vi "Main.vi"(11 "Module Admin":refnum<class "Delacor_lib_QMH_Module Admin.lvclass">) -> ()   [LabVIEW 2020, in "Molde.lvlib"]
doc: "This template is based off of the Queued Message Handler design pattern and the Queued Message Handler project template that ships with LabVIEW.\n\nThe main difference is that the queue is private to this module and communication between modules is performed via Broadcast and Request events.\n\nRequest events are wrapped in public API methods and are handled in the Event Handling Loop (EHL) of this VI. Any module can register for Broadcast events sent by this module. The EHL generates messages based on user interface actions.\n\nThe Message Handling Loop (MHL) processes messages generated by the EHL, or by other messages. The messages are string values, so new messages can be added easily to the Message Cases case structure in the MHL. Each message cluster can also provide an optional value for Message Data, which is a variant that can be converted to whatever message-specific data is required.\n_____\nBased on Delacor QMH Project Template 5.0.0.82."
uses:
  Molde.lvlib
  <vilib>/Delacor/Delacor QMH/Libraries/Module Admin_class/Delacor_lib_QMH_Module Admin.lvclass
  Module Data--cluster.ctl
  <vilib>/Delacor/Delacor QMH/Libraries/Message Queue_class/Delacor_lib_QMH_Message Queue.lvclass/Delacor_lib_QMH_Message Queue.ctl
  Stop Argument--cluster.ctl
  <vilib>/Delacor/Delacor QMH/Libraries/Module Admin_class/Delacor_lib_QMH_Module Admin.lvclass/Delacor_lib_QMH_Module Admin.ctl
  <vilib>/Utility/miscctls.llb/LVPointTypeDef.ctl
  <vilib>/Delacor/Delacor QMH/Libraries/Message Queue_class/Delacor_lib_QMH_Enqueue Message (Single).vi
  <vilib>/Delacor/Delacor QMH/Libraries/Module Admin_class/Delacor_lib_QMH_Get External Launch.vi
  <vilib>/Utility/error.llb/Error Cluster From Error Code.vi
  <vilib>/ErrorRing/Error Ring.xnode
  <vilib>/Delacor/Delacor QMH/Libraries/Message Queue_class/Delacor_lib_QMH_Message Queue.lvclass
  Numpad/Numpad.lvlib
panel:
  in  "Insertar Subpanel NumPad":bool
  in  "Simulate MHL Error":bool
  in  "Simulate EHL Error":bool
  out "error out":errorcluster
  out "Status":string
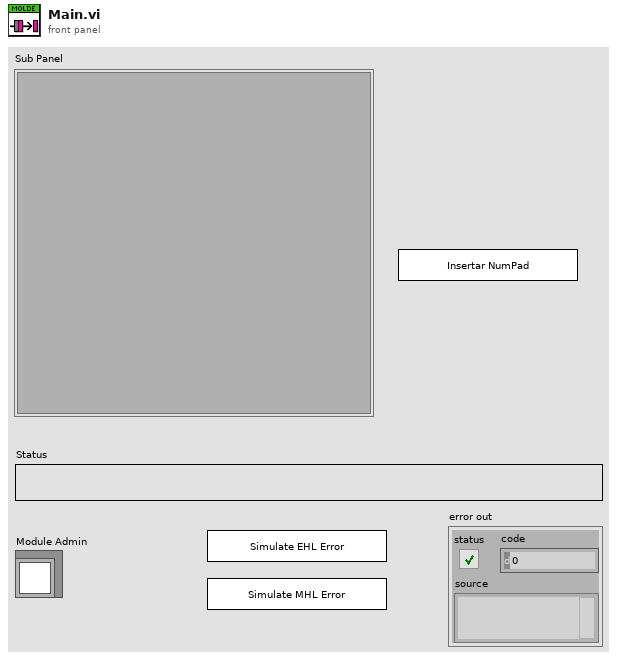
[diagram p1: front panel]
types:
  T1 = typedef "Molde.lvlib/Request Events--cluster.ctl" = cluster{"Stop Module":refnum<user-event>, "Show Panel":refnum<user-event>, "Hide Panel":refnum<user-event>, "Get Module Execution Status":refnum<user-event>, "Show Diagram":refnum<user-event>}
  T2 = typedef "Numpad.lvlib/Broadcast Events--cluster.ctl" = cluster{"Module Did Init":refnum<user-event>, "Status Updated":refnum<user-event>, "Error Reported":refnum<user-event>, "Module Did Stop":refnum<user-event>, "Update Module Execution Status":refnum<user-event>}
  T3 = typedef "Molde.lvlib/Module Data--cluster.ctl" = cluster{"Status":string}
  T4 = enum32{"invalid lock state", "Not Locked", "Locked (No Password)", "Password-protected"}
  T5 = typedef "Molde.lvlib/Stop Argument--cluster.ctl" = cluster{"Origin":string, "Exit via Stop Module Req?":bool, "Wait for Module to stop?":bool}
  T6 = typedef "LVPointTypeDef.ctl" = cluster{"Horizontal":i16, "Vertical":i16}
  T7 = enum32{"Invalid", "Standard", "Closed", "Hidden", "Minimized", "Maximized"}
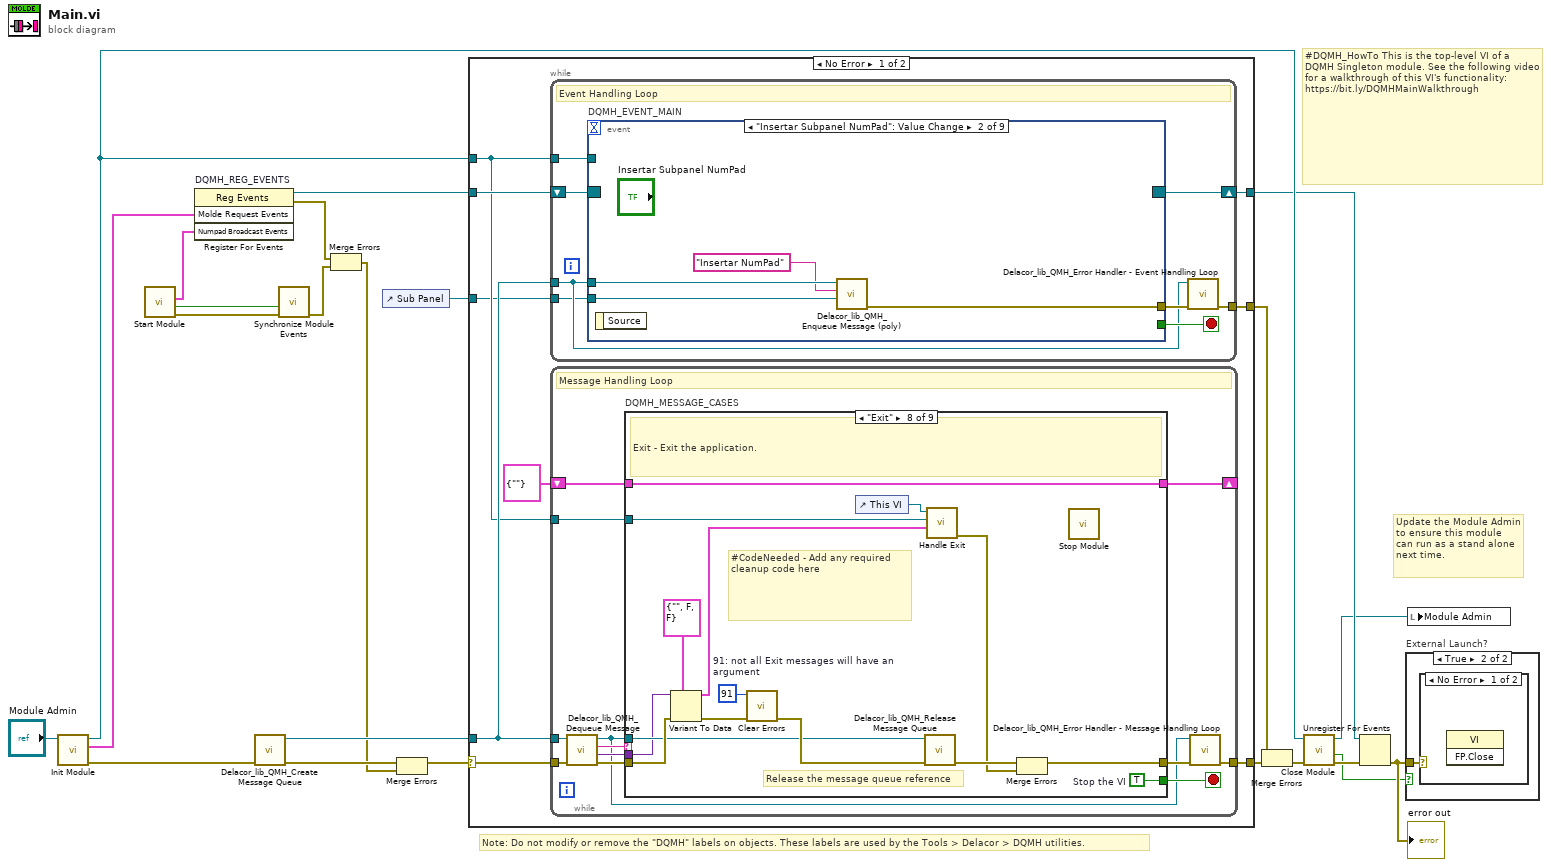
[diagram p0: block diagram]
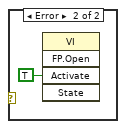
[diagram p3: hidden frame]
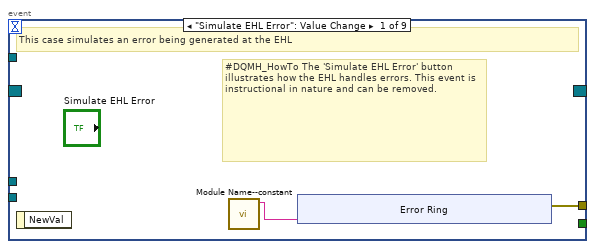
[diagram p4: hidden frame]
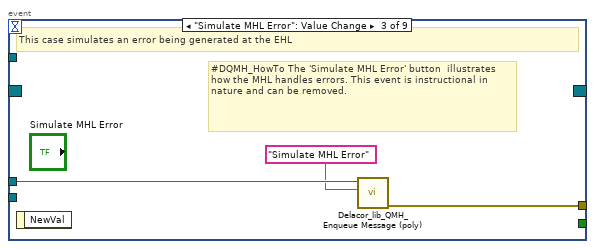
[diagram p5: hidden frame]
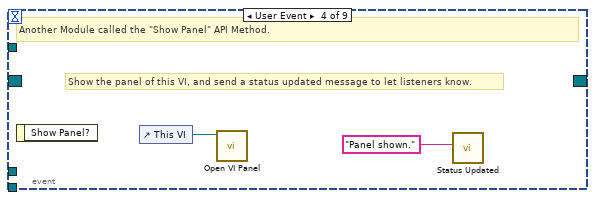
[diagram p6: hidden frame]
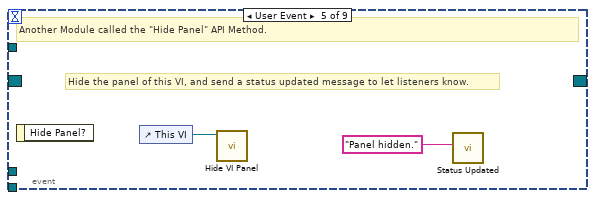
[diagram p7: hidden frame]
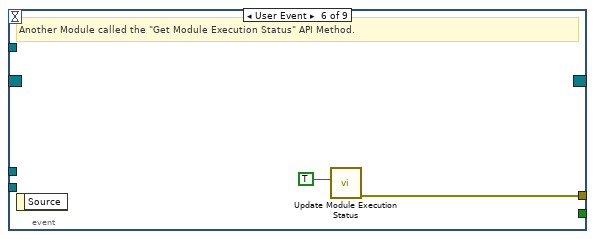
[diagram p8: hidden frame]
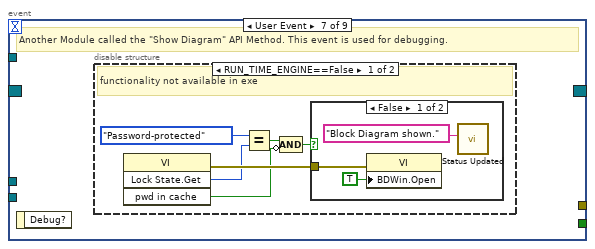
[diagram p9: hidden frame]
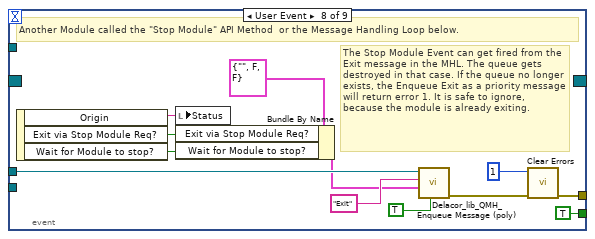
[diagram p12: hidden frame]
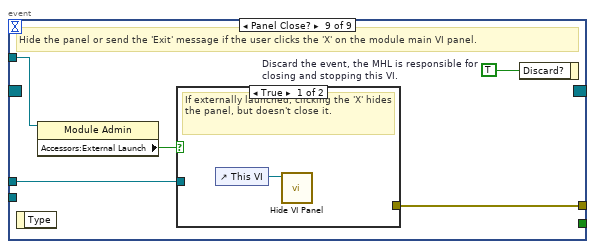
[diagram p13: hidden frame]
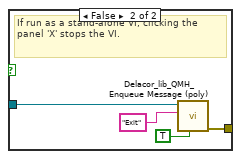
[diagram p14: hidden frame]
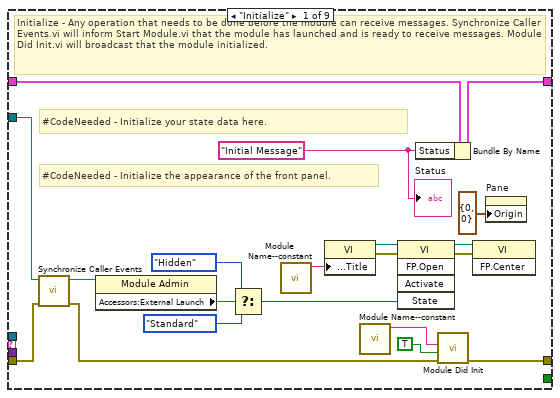
[diagram p15: hidden frame]
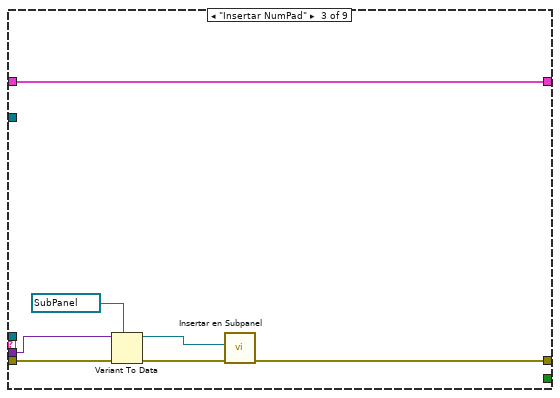
[diagram p17: hidden frame]
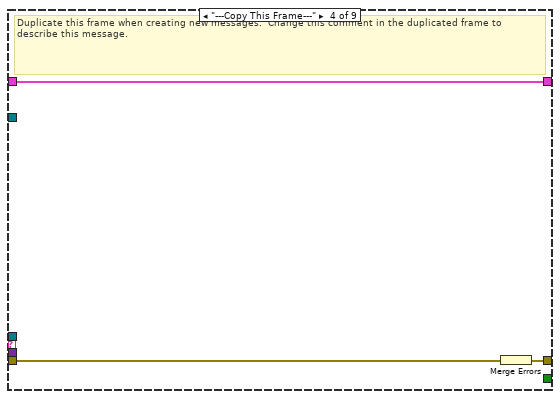
[diagram p18: hidden frame]
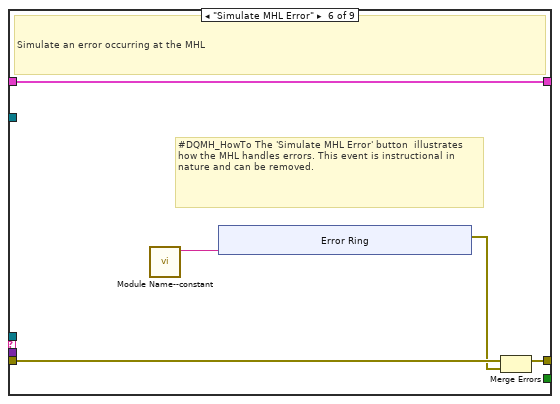
[diagram p20: hidden frame]
diagram:
  # "#DQMH_HowTo This is the top-level VI of a DQMH Singleton module. See the following video for a walkthrough of this VI's functionality: https://bit.ly/DQMHMainWalkthrough"
  # "Note: Do not modify or remove the \"DQMH\" labels on objects. These labels are used by the Tools > Delacor > DQMH utilities."
  # "Update the Module Admin to ensure this module can run as a stand alone next time."
  n1 = call "Init Module.vi"("Singleton Module Admin in"="Module Admin") -> ("error out"=w22:errorcluster, "Molde Request Events"=w12:T1, "Singleton Module Admin out"=w15:refnum<class "Delacor_lib_QMH_Module Admin.lvclass">)  [unwired: 8 in]
  n2 = call "Start Module.vi"() -> ("error out"=w5:errorcluster, "Wait for Event Sync?"=w7:bool, "Numpad Broadcast Events"=w6:T2)  [unwired: 8 in, 1 out]
  n3 = register-events "DQMH_REG_EVENTS"(w12, w6) -> (reference out=w13:refnum<event-registration>, error out=w4:errorcluster)  [unwired: 2 in]
  n4 = call <vilib>:"Delacor_lib_QMH_Create Message Queue.vi"("error in (no error)"=w22) -> ("error out"=w17:errorcluster, "Message Queue"=w11:refnum<class "Delacor_lib_QMH_Message Queue.lvclass">)  [unwired: 9 in]
  n5 = call "Synchronize Module Events.vi"("error in (no error)"=w5, "Wait for Event Sync?"=w7) -> ("error out"=w3:errorcluster)  [unwired: 9 in]
  n6 = Merge Errors(w4, w3) -> (w2:errorcluster)
  n7 = control-ref of="Sub Panel"() -> (w1:refnum<vi>)
  n8 = Merge Errors(w17, w2) -> (w16:errorcluster)
  n9 = case shown="No Error" w16 {
    selector: w16 -> [w30 w200]
    tunnel: [w32 w199] -> w23
    tunnel: [w29 w205] -> w14
    tunnel: w13 -> [w27 w205]
    tunnel: w11 -> [w26 w198]
    tunnel: [w31 _] -> w20
    tunnel: w15 -> [w25 w201]
    tunnel: w1 -> [w24 _]
    frame No Error {
      n10 = while {
        tunnel: w26 -> [w34]
        shift-right: [w37] -> w29
        shift-left: w27 -> [w38]
        tunnel: [w39] -> w31
        tunnel: w25 -> [w35]
        tunnel: w24 -> [w33]
        stop <- w36 stop-if-true
        # "Event Handling Loop"
        n11 = event "DQMH_EVENT_MAIN" shown="[1] \"Insertar Subpanel NumPad\": Value Change" {
          selector: w38 -> [_ _ _ _ _ _ _ _ _]
          dyn-events: [_ _ _ _ _ _ _ _ _] -> w37
          timeout: _ -> [_ _ _ _ _ _ _ _ _]
          tunnel: [_ _ _ _ _ _ _ TRUE ("Discard?") _] -> w36
          tunnel: w34 -> [_ w53 w55 _ _ _ _ w79 w86]
          tunnel: [w42 w50 w56 _ _ w62 _ w82 w88] -> w40
          tunnel: w35 -> [_ _ _ _ _ _ _ _ w85]
          tunnel: w33 -> [_ w52 _ _ _ _ _ _ _]
          event "Simulate EHL Error": Value Change {
            # "#DQMH_HowTo The 'Simulate EHL Error' button  illustrates how the EHL handles errors. This event is instructional in nature and can be removed."
            # "This case simulates an error being generated at the EHL"
            n12 = event-data() -> ()  [unwired: 1 in, 1 out]
            n13 = call "Module Name--constant.vi"() -> ("Module Name"=w41:string)  [unwired: 11 in]
            n14 = xnode "Error Ring"("parameter 0"=w41) -> ("error out"=w42:errorcluster)
          }
          event "Insertar Subpanel NumPad": Value Change {
            n15 = event-data() -> ()  [unwired: 1 in, 1 out]
            n16 = call-poly <vilib>:"Delacor_lib_QMH_Enqueue Message (poly).vi"("Message Data"=w52, "Message"="Insertar NumPad", "Message Queue in"=w53) -> ("error out"=w50:errorcluster)  [unwired: 7 in, 1 out]
          }
          event "Simulate MHL Error": Value Change {
            # "#DQMH_HowTo The 'Simulate MHL Error' button  illustrates how the MHL handles errors. This event is instructional in nature and can be removed."
            # "This case simulates an error being generated at the EHL"
            n17 = event-data() -> ()  [unwired: 1 in, 1 out]
            n18 = call-poly <vilib>:"Delacor_lib_QMH_Enqueue Message (poly).vi"("Message"="Simulate MHL Error", "Message Queue in"=w55) -> ("error out"=w56:errorcluster)  [unwired: 8 in, 1 out]
          }
          event User Event {
            # "Show the panel of this VI, and send a status updated message to let listeners know."
            # "Another Module called the \"Show Panel\" API Method."
            n19 = event-data() -> ()  [unwired: 1 in, 1 out]
            n20 = control-ref of="This VI"() -> (w58:refnum<vi>)
            n21 = call "Open VI Panel.vi"("VI"=w58) -> ()  [unwired: 10 in, 1 out]
            n22 = call "Status Updated.vi"("Status"="Panel shown." ("format string")) -> ()  [unwired: 10 in, 1 out]
          }
          event User Event {
            # "Hide the panel of this VI, and send a status updated message to let listeners know."
            # "Another Module called the \"Hide Panel\" API Method."
            n23 = event-data() -> ()  [unwired: 1 in, 1 out]
            n24 = control-ref of="This VI"() -> (w60:refnum<vi>)
            n25 = call "Hide VI Panel.vi"("VI"=w60) -> ()  [unwired: 10 in, 1 out]
            n26 = call "Status Updated.vi"("Status"="Panel hidden." ("format string")) -> ()  [unwired: 10 in, 1 out]
          }
          event User Event {
            # "Another Module called the \"Get Module Execution Status\" API Method."
            n27 = event-data() -> ()  [unwired: 1 in, 1 out]
            n28 = call "Update Module Execution Status.vi"("Running?"=TRUE) -> ("error out"=w62:errorcluster)  [unwired: 10 in]
          }
          event User Event {
            # "Another Module called the \"Show Diagram\" API Method. This event is used for debugging."
            n29 = event-data() -> ()  [unwired: 1 in, 1 out]
            n30 = disable-structure shown="RUN_TIME_ENGINE==False" {
              frame condition #0 (active) {
                # "functionality not available in exe"
                n31 = invoke class="VI" method="Lock State.Get"() -> (error out=w68:errorcluster, "Get Lock State"=w67:T4, "pwd in cache"=w64:bool)  [unwired: 4 in, 1 out]
                n32 = Equal?(x=T4."Password-protected", y=w67) -> (x = y?=w65:bool)
                n33 = Compound Arithmetic op=AND(w65, invert w64) -> (w63:bool)
                n34 = case shown="False" w63 {
                  tunnel: w68 -> [w71 _]
                  frame False {
                    n35 = property class="VI"(error in=w71, "BDWin.Open"=TRUE ("Block Diagram Window:Open")) -> ()  [unwired: 1 in, 2 out]
                    n36 = call "Status Updated.vi"("Status"="Block Diagram shown." ("format string")) -> ()  [unwired: 10 in, 1 out]
                  }
                  frame True {
                    # "Password-protected VI, and the password is not in the cache. Do not show the diagram."
                  }
                }
              }
              frame condition #1 {
              }
            }
          }
          event User Event {
            # "The Stop Module Event can get fired from the Exit message in the MHL. The queue gets destroyed in that case. If the queue no longer exists, the Enqueue Exit as a priority message will return error 1. It is safe to ignore, because the module is already exiting."
            # "Another Module called the \"Stop Module\" API Method  or the Message Handling Loop below."
            n37 = event-data() -> ("Origin"=w78:string, "Exit via Stop Module Req?"=w74:bool, "Wait for Module to stop?"=w73:bool)  [unwired: 1 in]
            n38 = local write "Status"(w78) -> ()
            n39 = Bundle By Name(cluster=T5 {"Origin"="", "Exit via Stop Module Req?"=FALSE, "Wait for Module to stop?"=FALSE} ("Stop Argument"), "Exit via Stop Module Req?"=w74, "Wait for Module to stop?"=w73) -> (w72:T5)
            n40 = call-poly <vilib>:"Delacor_lib_QMH_Enqueue Message (poly).vi"("Priority Message? (F)"=TRUE, "Message Data"=w72, "Message"="Exit", "Message Queue in"=w79) -> ("error out"=w83:errorcluster)  [unwired: 6 in, 1 out]
            n41 = call <vilib>:"Clear Errors.vi"("error in (no error)"=w83, "specific error code to clear (0: all)"=1) -> ("error out"=w82:errorcluster)  [unwired: 4 in, 1 out]
          }
          event Panel Close? {
            w87 = TRUE  # Discard the event, the MHL is responsible for closing and stopping this VI.
            # "Hide the panel or send the 'Exit' message if the user clicks the 'X' on the module main VI panel."
            n42 = event-data() -> ()  [unwired: 1 in, 1 out]
            n43 = property class="Module Admin"(reference=w85) -> ("Accessors:External Launch"=w84:bool)  [unwired: 1 in, 2 out]
            n44 = case shown="True" w84 {
              tunnel: w86 -> [_ w92]
              tunnel: [_ w93] -> w88
              frame True {
                # "If externally launched, clicking the 'X' hides the panel, but doesn't close it."
                n45 = control-ref of="This VI"() -> (w89:refnum<vi>)
                n46 = call "Hide VI Panel.vi"("VI"=w89) -> ()  [unwired: 10 in, 1 out]
              }
              frame False {
                # "If run as a stand-alone VI, clicking the panel 'X' stops the VI."
                n47 = call-poly <vilib>:"Delacor_lib_QMH_Enqueue Message (poly).vi"("Priority Message? (F)"=TRUE, "Message"="Exit", "Message Queue in"=w92) -> ("error out"=w93:errorcluster)  [unwired: 7 in, 1 out]
              }
            }
            n48 = event-data("Discard?"=w87) -> ()  [unwired: 1 in, 1 out]
          }
        }
        n49 = call-dynamic "Delacor_lib_QMH_Error Handler - Event Handling Loop.vi"("error in (no error)"=w40, "Message Queue in"=w34) -> ("dup error in"=w39:errorcluster)  [unwired: 8 in, 1 out]
      }
      n50 = while {
        tunnel: w26 -> [w96]
        shift-right: [w100] -> _
        shift-left: T3 {"Status"=""} ("Data Cluster") -> [w101]
        tunnel: w30 -> [w104]
        tunnel: [w102] -> w32
        tunnel: w25 -> [w94]
        stop <- w99 stop-if-true
        # "Message Handling Loop"
        n51 = call-dynamic "Delacor_lib_QMH_Dequeue Message.vi"("error in (no error)"=w104, "Message Queue in"=w96) -> ("error out"=w103:errorcluster, "Message Data"=w97:variant, "Message"=w98:string, "Message Queue out"=w95:refnum<class "Delacor_lib_QMH_Message Queue.lvclass">)  [unwired: 6 in]
        n52 = case "DQMH_MESSAGE_CASES" shown="\"Exit\"" w98 {
          selector: w98 -> [_ _ _ _ _ _ _ _ w185]
          tunnel: w95 -> [_ _ _ _ _ _ w155 w177 _]
          tunnel: w103 -> [w123 w127 w134 w137 w139 w144 w162 w183 w187]
          tunnel: [w121 w127 w128 w136 w139 w143 w158 w180 w188] -> w105
          tunnel: w101 -> [w112 w126 w133 w135 w138 w141 w157 w176 w186]
          tunnel: [w111 w126 w133 w135 w138 w141 w157 w176 w186] -> w100
          tunnel: [_ _ _ _ _ _ _ w175 _] -> w99
          tunnel: w97 -> [_ _ w132 _ _ _ w156 w174 _]
          tunnel: w94 -> [w113 _ _ _ _ _ w154 w169 _]
          frame "Initialize" {
            w106 = "Initial Message" ("Initial Message")
            # "#CodeNeeded - Initialize the appearance of the front panel."
            # "#CodeNeeded - Initialize your state data here."
            # "Initialize - Any operation that needs to be done before the module can receive messages. Synchronize Caller Events.vi will inform Start Module.vi that the module has launched and is ready to receive messages. Module Did Init.vi will broadcast that the module initialized."
            n53 = call "Synchronize Caller Events.vi"("error in (no error)"=w123, "Singleton Module Admin in"=w113) -> ("error out"=w122:errorcluster, "Singleton Module Admin out"=w108:refnum<class "Delacor_lib_QMH_Module Admin.lvclass">)  [unwired: 8 in]
            n54 = property class="Module Admin"(reference=w108) -> ("Accessors:External Launch"=w117:bool)  [unwired: 1 in, 2 out]
            n55 = Select(t=T7."Hidden" ("State"), s=w117, f=T7."Standard" ("State")) -> (s? t:f=w114:T7)
            n56 = call "Module Name--constant.vi"() -> ("Module Name"=w120:string)  [unwired: 11 in]
            n57 = property class="VI"("Front Panel.Title"=w120) -> (reference out=w119:refnum<vi>, error out=w125:errorcluster)  [unwired: 2 in]
            n58 = call "Module Name--constant.vi"() -> ("Module Name"=w109:string)  [unwired: 11 in]
            n59 = invoke class="VI" method="FP.Open"(reference=w119, error in=w125, "State"=w114) -> (reference out=w118:refnum<vi>, error out=w124:errorcluster)  [unwired: 2 in, 3 out]
            n60 = Bundle By Name(cluster=w112, "Status"=w106) -> (w111:T3)
            n61 = call "Module Did Init.vi"("error in (no error)"=w122, "Initialized?"=TRUE, "Origin"=w109) -> ("error out"=w121:errorcluster)  [unwired: 8 in]
            n62 = invoke class="VI" method="FP.Center"(reference=w118, error in=w124) -> ()  [unwired: 1 in, 3 out]
            n63 = property on="Pane" class="Pane"("Origin"=T6 {"Horizontal"=0, "Vertical"=0}) -> ()  [unwired: 2 in, 2 out]
            "Status" <- w106
          }
          frame "--- Module Specific ---" {
            # "Separator -- The following cases handle messages specific to this Module."
          }
          frame "Insertar NumPad" {
            n64 = Variant To Data(error in=w134, type=refnum<vi> refnum ("Sub Panel"), Variant=w132) -> (data=w130:refnum<vi>, error out=w129:errorcluster)
            n65 = call "Insertar en Subpanel.vi"("error in (no error)"=w129, "Subpanel Ref"=w130) -> ("error out"=w128:errorcluster)  [unwired: 9 in]
          }
          frame "---Copy This Frame---" {
            # "Duplicate this frame when creating new messages.  Change this comment in the duplicated frame to describe this message."
            n66 = Merge Errors(w137) -> (w136:errorcluster)
          }
          frame "--- Exit and Error Handling---" {
            # "Separator - The following cases handle errors and exit messages."
          }
          frame "Simulate MHL Error" {
            # "#DQMH_HowTo The 'Simulate MHL Error' button  illustrates how the MHL handles errors. This event is instructional in nature and can be removed."
            # "Simulate an error occurring at the MHL"
            n67 = call "Module Name--constant.vi"() -> ("Module Name"=w140:string)  [unwired: 11 in]
            n68 = xnode "Error Ring"("parameter 0"=w140) -> ("error out"=w142:errorcluster)
            n69 = Merge Errors(w144, w142) -> (w143:errorcluster)
          }
          frame "Error" {
            # "#CodeRecommended - If you ever change the name of this \"Error\" message, you'll need to update the name in the Check Loop Error.vi as well."
            # "#CodeRecommended - If the module is running in standalone mode (External Launch = FALSE), this code will pop up an error dialog and call the 'Exit' message if an error occurs. Add more fine-grained error handling here."
            # "Error - Check the error message data and respond accordingly. This message is sent by the \"Error Handler\" VIs at the end of each loop in this application."
            n70 = property class="Module Admin"(reference=w154) -> ("Accessors:External Launch"=w153:bool)  [unwired: 1 in, 2 out]
            n71 = Variant To Data(error in=w162, type=errorcluster {"status"=FALSE, "code"=0, "source"=""} ("error constant"), Variant=w156) -> (data=w163:errorcluster, error out=w160:errorcluster)
            n72 = call "Module Name--constant.vi"() -> ("Module Name"=w152:string)  [unwired: 11 in]
            n73 = call "Error Reported.vi"("Additional Information"=w152, "Error"=w163) -> ()  [unwired: 9 in, 1 out]
            n74 = case shown="False" w153 {
              tunnel: [w168 _] -> w159
              tunnel: w155 -> [w166 _]
              tunnel: w163 -> [w167 _]
              frame False {
                # "If the module is running standalone, then pop up an error dialog and call the \"Exit\" message."
                n75 = call <vilib>:"Simple Error Handler.vi"("error in (no error)"=w167) -> ()  [unwired: 4 in, 5 out]
                n76 = call-poly <vilib>:"Delacor_lib_QMH_Enqueue Message (poly).vi"("Priority Message? (F)"=TRUE, "Message"="Exit", "Message Queue in"=w166) -> ("error out"=w168:errorcluster)  [unwired: 7 in, 1 out]
              }
              frame True {
                # "If the module was launched externally, calling the Error Reported broadcast VI is the only action performed by the \"Error\" message. The module's caller can then process the error appropriately."
              }
            }
            n77 = Merge Errors(w160, w159) -> (w158:errorcluster)
            n78 = local write "error out"(w158) -> ()
          }
          frame "Exit" {
            w173 = 91  # 91: not all Exit messages will have an argument
            w175 = TRUE  # Stop the VI
            # "Release the message queue reference"
            # "#CodeNeeded - Add any required cleanup code here"
            # "Exit - Exit the application."
            n79 = Variant To Data(error in=w183, type=T5 {"Origin"="", "Exit via Stop Module Req?"=FALSE, "Wait for Module to stop?"=FALSE} ("Stop Argument"), Variant=w174) -> (data=w171:T5, error out=w179:errorcluster)
            n80 = call <vilib>:"Clear Errors.vi"("error in (no error)"=w179, "specific error code to clear (0: all)"=w173) -> ("error out"=w182:errorcluster)  [unwired: 4 in, 1 out]
            n81 = control-ref of="This VI"() -> (w170:refnum<vi>)
            n82 = call-dynamic "Delacor_lib_QMH_Release Message Queue.vi"("error in (no error)"=w182, "Message Queue"=w177) -> ("error out"=w181:errorcluster)  [unwired: 9 in]
            n83 = call "Handle Exit.vi"("Stop Argument"=w171, "Admin in"=w169, "VI reference"=w170) -> ("error out"=w178:errorcluster)  [unwired: 7 in, 1 out]
            n84 = Merge Errors(w181, w178) -> (w180:errorcluster)
            n85 = call "Stop Module.vi"() -> ()  [unwired: 11 in, 1 out]
          }
          frame Default {
            # "'Default' case only runs if there is a message that isn't defined in any of the other cases.  Output a programming error."
            n86 = call "Module Name--constant.vi"() -> ("Module Name"=w184:string)  [unwired: 11 in]
            n87 = xnode "Error Ring"("parameter 0"=w185, "parameter 1"=w184) -> ("error out"=w189:errorcluster)
            n88 = Merge Errors(w187, w189) -> (w188:errorcluster)
          }
        }
        n89 = call-dynamic "Delacor_lib_QMH_Error Handler - Message Handling Loop.vi"("error in (no error)"=w105, "Message Queue in"=w95) -> ("dup error in"=w102:errorcluster)  [unwired: 8 in, 1 out]
      }
    }
    frame Error {
      # "Synchronize Caller Events.vi will inform Start Module.vi that the module has launched and will let the code calling Start Module.vi register for broadcasts and would permit the caller receive the broadcast that an error occurred at launch time."
      n90 = call-dynamic "Delacor_lib_QMH_Release Message Queue.vi"("error in (no error)"=w200, "Message Queue"=w198) -> ("error out"=w199:errorcluster)  [unwired: 9 in]
      n91 = call "Synchronize Caller Events.vi"("Singleton Module Admin in"=w201) -> ("error out"=w206:errorcluster)  [unwired: 9 in, 1 out]
      n92 = call "Module Name--constant.vi"() -> ("Module Name"=w204:string)  [unwired: 11 in]
      n93 = Format Into String(format string="An error occurred during initialization. %s is no longer running.", w204) -> (resulting string=w202:string)  [unwired: 2 in, 1 out]
      n94 = Merge Errors(w199, w206) -> (w207:errorcluster)
      n95 = call "Error Reported.vi"("Additional Information"=w202, "Error"=w207) -> ()  [unwired: 9 in, 1 out]
    }
  }
  n96 = Merge Errors(w20, w23) -> (w19:errorcluster)
  n97 = call "Close Module.vi"("error in (no error)"=w19, "Module Admin in"=w15) -> ("error out"=w21:errorcluster, "External Launch"=w8:bool, "Module Admin out"=w9:refnum<class "Delacor_lib_QMH_Module Admin.lvclass">)  [unwired: 7 in]
  n98 = Unregister For Events(event registration refnum=w14, error in=w21) -> (error out=w18:errorcluster)
  "error out" <- w18
  n99 = case "External Launch?" shown="True" w8 {
    tunnel: w18 -> [_ w208]
    frame False {
    }
    frame True {
      n100 = case shown="No Error" w208 {
        frame No Error {
          n101 = invoke class="VI" method="FP.Close"() -> ()  [unwired: 3 in, 3 out]
        }
        frame Error {
          n102 = invoke class="VI" method="FP.Open"("Activate"=TRUE ("Activate?")) -> ()  [unwired: 4 in, 5 out]
        }
      }
    }
  }
  n103 = local write "Module Admin"(w9) -> ()
